vi "updateCellPositionsBasedOnNewStageZero.vi"(8 "error in":errorcluster, 9 "preZeroStageCooridinates":i32[](array[numeric]), 10 "transform cluster + actuator":T1, 11 "common cluster":T2) -> (0 "error out":errorcluster)   [LabVIEW 2015]
uses:
  pipette cleaning/pressure box/cleaning_soft/controls/actuator_type.ctl
  pipette cleaning/pressure box/cleaning_soft/controls/actuator_cluster.ctl
  machine_vision/coordinate model vis/transform_properties_actuators.ctl
  machine_vision/controls/transform_cluster_actuator.ctl
  controls/NH_method.ctl
  pipette cleaning/pressure box/cleaning_soft/controls/pressure_box_type.ctl
  pipette cleaning/pressure box/cleaning_soft/controls/pressure_box_control.ctl
  multipatch/controls/multipatch_common_controls_v4.ctl
panel:
  # "Stage:"
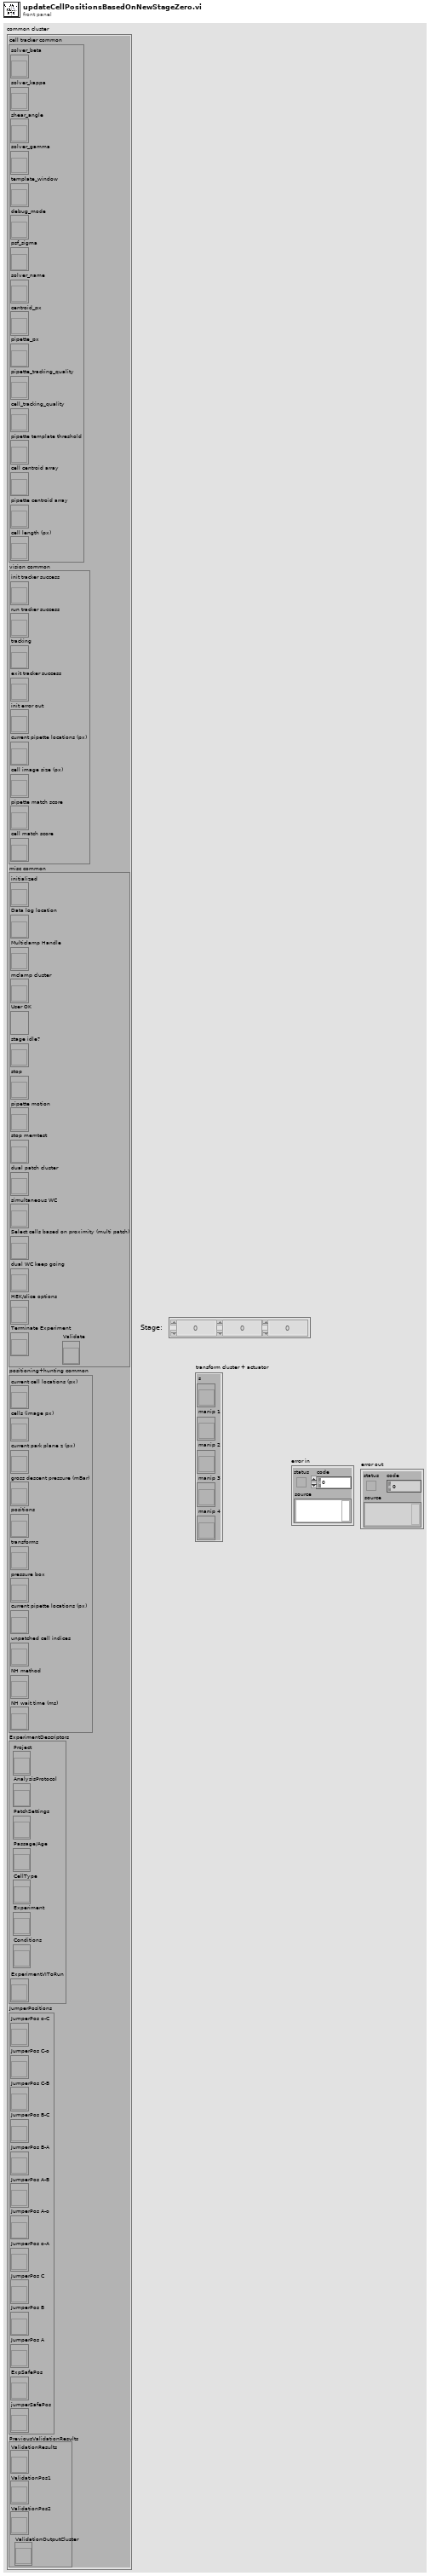
[diagram p1: front panel]
types:
  T1 = typedef "transform_cluster_actuator.ctl" = cluster{"s":refnum<vi>, "manip 1":refnum<vi>, "manip 2":refnum<vi>, "manip 3":refnum<vi>, "manip 4":refnum<vi>}
  T2 = typedef "multipatch_common_controls_v4.ctl" = cluster{"cell tracker common":cluster{"solver_beta":refnum<vi>, "solver_kappa":refnum<vi>, "shear_angle":refnum<vi>, "solver_gamma":refnum<vi>, "template_window":refnum<vi>, "debug_mode":refnum<vi>, "psf_sigma":refnum<vi>, "solver_name":refnum<vi>, "centroid_px":refnum<vi>, "pipette_px":refnum<vi>, "pipette_tracking_quality":refnum<vi>, "cell_tracking_quality":refnum<vi>, "pipette template threshold":refnum<vi>, "cell centroid array":refnum<vi>, "pipette centroid array":refnum<vi>, "cell length (px)":refnum<vi>}, "vision common":cluster{"init tracker success":refnum<vi>, "run tracker success":refnum<vi>, "tracking":refnum<vi>, "exit tracker success":refnum<vi>, "init error out":refnum<vi>, "current pipette locations (px)":refnum<vi>, "cell image size (px)":refnum<vi>, "pipette match score":refnum<vi>, "cell match score":refnum<vi>}, "misc common":cluster{"initialized":refnum<vi>, "Data log location":refnum<vi>, "Multiclamp Handle":refnum<vi>, "mclamp cluster":refnum<vi>, "User OK":refnum<vi>, "stage idle?":refnum<vi>, "stop":refnum<vi>, "pipette motion":refnum<vi>, "stop memtest":refnum<vi>, "dual patch cluster":refnum<vi>, "simultaneous WC":refnum<vi>, "Select cells based on proximity (multi patch)":refnum<vi>, "dual WC keep going":refnum<vi>, "HEK/slice options":refnum<vi>, "Terminate Experiment":refnum<vi>, "Validate":refnum<vi>}, "positioning+hunting common":cluster{"current cell locations (px)":refnum<vi>, "cells (image px)":refnum<vi>, "current park plane z (px)":refnum<vi>, "gross descent pressure (mBar)":refnum<vi>, "positions":refnum<vi>, "transforms":refnum<vi>, "pressure box":refnum<vi>, "current pipette locations (px)":refnum<vi>, "unpatched cell indices":refnum<vi>, "NH method":refnum<vi>, "NH wait time (ms)":refnum<vi>}, "ExperimentDescriptors":cluster{"Project":refnum<vi>, "AnalysisProtocol":refnum<vi>, "PatchSettings":refnum<vi>, "Passage/Age":refnum<vi>, "CellType":refnum<vi>, "Experiment":refnum<vi>, "Conditions":refnum<vi>, "ExperimentVIToRun":refnum<vi>}, "JumperPositions":cluster{"JumperPos o-C":refnum<vi>, "JumperPos C-o":refnum<vi>, "JumperPos C-B":refnum<vi>, "JumperPos B-C":refnum<vi>, "JumperPos B-A":refnum<vi>, "JumperPos A-B":refnum<vi>, "JumperPos A-o":refnum<vi>, "JumperPos o-A":refnum<vi>, "JumperPos C":refnum<vi>, "JumperPos B":refnum<vi>, "JumperPos A":refnum<vi>, "ExpSafePos":refnum<vi>, "jumperSafePos":refnum<vi>}, "PreviousValidationResults":cluster{"ValidationResults":refnum<vi>, "ValidationPos1":refnum<vi>, "ValidationPos2":refnum<vi>, "ValidationOutputCluster":refnum<vi>}}
  T3 = typedef "transform_properties_actuators.ctl" = cluster{"theta (deg)":dbl, "X sc factor (px/step)":dbl, "Y sc factor (px/step)":dbl, "zero loc (x,y,z)":dbl[], "flip y?":bool, "flip x?":bool, "gamma (deg)":dbl, "flip z?":bool, "Z sc factor (px/step)":dbl, "actuator":T4, "safe space (steps)":i32[]}
  T4 = typedef "actuator_cluster.ctl" = cluster{"Actuator COM":refnum<visa-resource-name>, "Actuator type":T5}
  T5 = typedef "actuator_type.ctl" = enum16{"Scientifica", "Sutter", "Demo", "Off"}
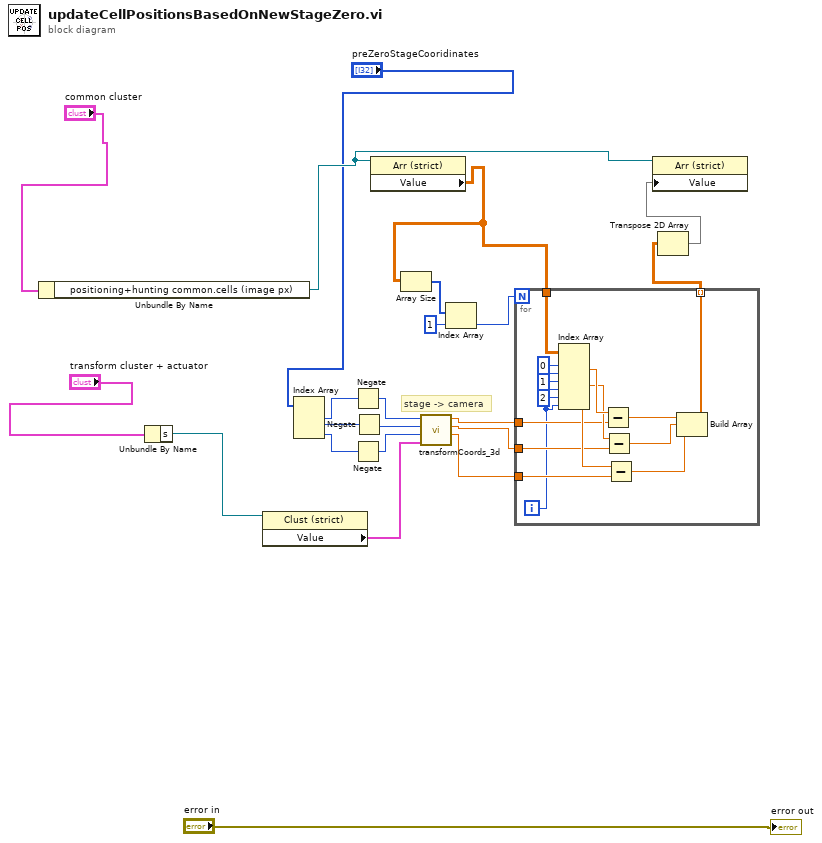
[diagram p0: block diagram]
diagram:
  # "stage -> camera"
  n1 = Unbundle By Name("common cluster") -> ("positioning+hunting common.cells (image px)"=w22:refnum<vi>)
  n2 = Unbundle By Name("transform cluster + actuator") -> ("s"=w15:refnum<vi>)
  n3 = property class="Clust (strict)"(reference=w15) -> ("Value"=w14:T3)  [unwired: 1 in, 2 out]
  n4 = Index Array(array="preZeroStageCooridinates") -> (element #1=w12:i32, element #2=w9:i32, element #3=w8:i32)  [unwired: 3 in]
  n5 = Negate(x=w12) -> (-x=w11:i32)
  n6 = Negate(x=w8) -> (-x=w7:i32)
  n7 = Negate(x=w9) -> (-x=w10:i32)
  n8 = property class="Arr (strict)"(reference=w22) -> ("Value"=w6:dbl[][])  [unwired: 1 in, 2 out]
  n9 = Array Size(array=w6) -> (size(s)=w5:i32[])
  n10 = call "transformCoords_3d.vi"("transform properties"=w14, "z"=w7, "y"=w10, "x"=w11) -> ("z out"=w18:dbl, "y out"=w17:dbl, "x out"=w19:dbl)  [unwired: 5 in]
  n11 = Index Array(array=w5, index=1) -> (element=w4:i32)
  n12 = for {
    N: w4 -> [_]
    tunnel: w6 -> [w37]
    tunnel: w19 -> [w33]
    tunnel: w18 -> [w32]
    tunnel: w17 -> [w31]
    tunnel: [w27] -> w2 mode=indexing
    i -> [w23]
    n13 = Index Array(array=w37, index (row) #1=0 ("disabled index (row)"), index (col) #1=w23, index (row) #2=1 ("disabled index (row)"), index (col) #2=w23, index (row) #3=2 ("index (row)"), index (col) #3=w23) -> (element #1=w36:dbl, element #2=w35:dbl, element #3=w34:dbl)
    n14 = Subtract(x=w36, y=w33) -> (x-y=w30:dbl)
    n15 = Subtract(x=w35, y=w31) -> (x-y=w29:dbl)
    n16 = Subtract(x=w34, y=w32) -> (x-y=w28:dbl)
    n17 = Build Array(w30, w29, w28) -> (w27:dbl[])
  }
  n18 = Transpose 2D Array(2D array=w2) -> (transposed array=w1:dbl[][])
  n19 = property class="Arr (strict)"(reference=w22, "Value"=w1) -> ()  [unwired: 1 in, 2 out]
  "error out" <- "error in"
